vi "Score Particles.vi"(8 "Area Size Limit":i32=444, 9 "Particle Count Limit":i32=10, 11 "Image Refnum in":T2) -> (0 "Size Array":T1(array[cluster]), 2 "Scored Particle Info":T3(array[cluster]), 3 "Image Refnum out":T2)   [LabVIEW 2011]
doc: "Score the largest particles in the image to determine how well they match the target attributes. Specifically, calculate how rectangular a particle is, inspect its aspect ratio, and determine if it is hollow (having pixels on around the edges, but off in the large center)."
uses:
  <vilib>/vision/Image Controls.llb/IMAQ Image.ctl
  <vilib>/vision/NI_Vision_Development_Module.lvlib
panel:
  out "Bounding Height":dbl
  out "Bounding Width":dbl
  out "Area":dbl
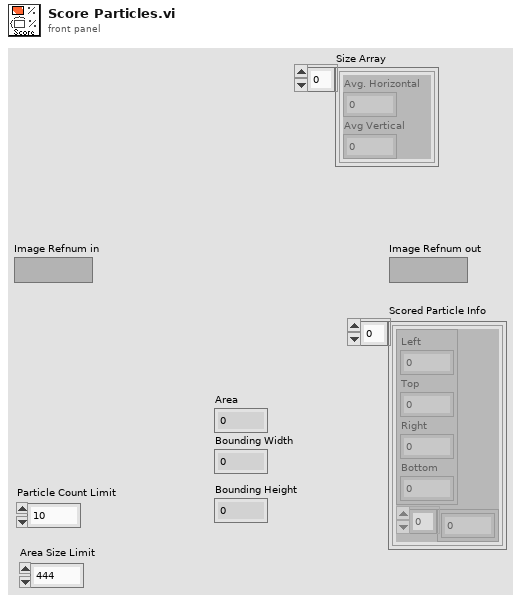
[diagram p1: front panel]
types:
  T1 = cluster{"Avg. Horizontal ":dbl, "Avg Vertical":dbl}[]
  T2 = typedef "IMAQ Image.ctl" = refnum<image>
  T3 = cluster{cluster{"Left":dbl, "Top":dbl, "Right":dbl, "Bottom":dbl}, dbl[]}[]
  T4 = typedef "Particle Parameters" = i32
  T5 = typedef "Image Type" = u32
  T6 = cluster{"Left":dbl, "Top":dbl, "Right":dbl, "Bottom":dbl}
  T7 = cluster{cluster{"Left":dbl, "Top":dbl, "Right":dbl, "Bottom":dbl}, dbl[]}
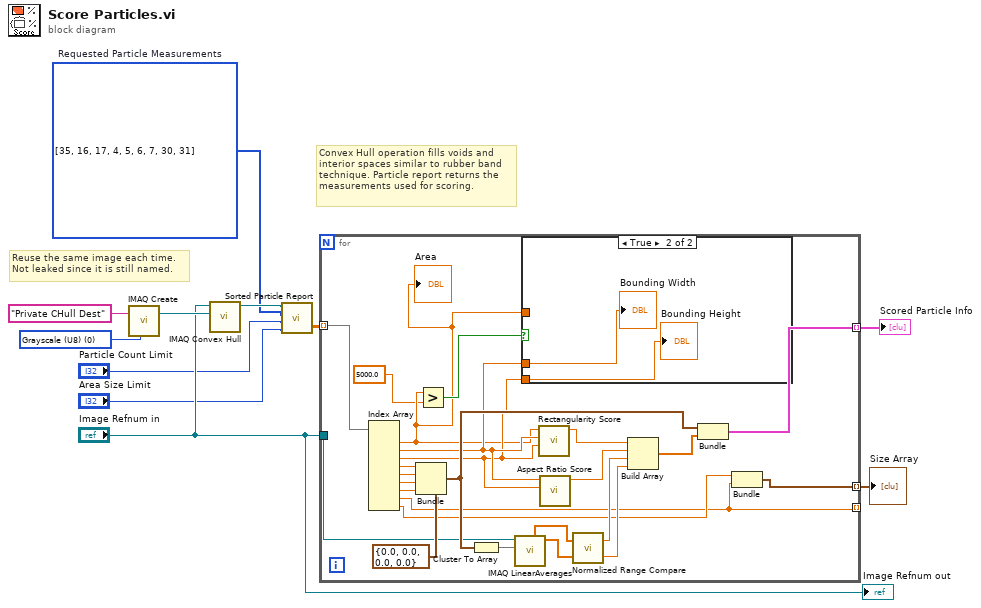
[diagram p0: block diagram]
diagram:
  w2 = T4[] [35, 16, 17, 4, 5, 6, 7, 30, 31] items=["Center of Mass X", "Center of Mass Y", "First Pixel X", "First Pixel Y", "Bounding Rect Left", "Bounding Rect Top", "Bounding Rect Right", "Bounding Rect Bottom", "Max Feret Diameter Start X", "Max Feret Diameter Start Y", "Max Feret Diameter End X", "Max Feret Diameter End Y", "Max Horiz. Segment Length Left", "Max Horiz. Segment Length Right", "Max Horiz. Segment Length Row", "-", "Bounding Rect Width", "Bounding Rect Height", "Bounding Rect Diagonal", "Perimeter", "Convex Hull Perimeter", "Holes' Perimeter", "Max Feret Diameter", "Equivalent Ellipse Major Axis", "Equivalent Ellipse Minor Axis", "Equivalent Ellipse Minor Axis (Feret)", "Equivalent Rect Long Side", "Equivalent Rect Short Side", "Equivalent Rect Diagonal", "Equivalent Rect Short Side (Feret)", "Average Horiz. Segment Length", "Average Vert. Segment Length", "Hydraulic Radius", "Waddel Disk Diameter", "-", "Area", "Holes' Area", "Particle & Holes' Area", "Convex Hull Area", "Image Area", "-", "Number of Holes", "Number of Horiz. Segments", "Number of Vert. Segments", "-", "Orientation", "Max Feret Diameter Orientation", "-", "% Area/Image Area", "% Area/(Particle & Holes' Area)", "Ratio of Equivalent Ellipse Axes", "Ratio of Equivalent Rect Sides", "-", "Elongation Factor", "Compactness Factor", "Heywood Circularity Factor", "Type Factor", "-", "Sum X", "Sum Y", "Sum XX", "Sum XY", "Sum YY", "Sum XXX", "Sum XXY", "Sum XYY", "Sum YYY", "-", "Moment of Inertia XX", "Moment of Inertia XY", "Moment of Inertia YY", "Moment of Inertia XXX", "Moment of Inertia XXY", "Moment of Inertia XYY", "Moment of Inertia YYY", "Norm. Moment of Inertia XX", "Norm. Moment of Inertia XY", "Norm. Moment of Inertia YY", "Norm. Moment of Inertia XXX", "Norm. Moment of Inertia XXY", "Norm. Moment of Inertia XYY", "Norm. Moment of Inertia YYY", "Hu Moment 1", "Hu Moment 2", "Hu Moment 3", "Hu Moment 4", "Hu Moment 5", "Hu Moment 6", "Hu Moment 7"]  # Requested Particle Measurements
  w9 = T5 0 items=["Grayscale (U8)", "Grayscale (I16)", "Grayscale (SGL)", "Complex (CSG)", "RGB (U32)", "HSL (U32)", "RGB (U64)", "Grayscale (U16)"] ("Image Type")
  # "Reuse the same image each time.\nNot leaked since it is still named."
  # "Convex Hull operation fills voids and\ninterior spaces similar to rubber band\ntechnique. Particle report returns the\nmeasurements used for scoring."
  n1 = call "IMAQ Create"("Image Name"="Private CHull Dest", "Image Type"=w9) -> ("New Image"=w8:T2)  [unwired: 2 in, 2 out]
  n2 = call "IMAQ Convex Hull"("Image Dst"=w8, "Image Src"="Image Refnum in") -> ("Image Dst Out"=w6:T2)  [unwired: 2 in, 7 out]
  n3 = call "Sorted Particle Report.vi"("Area Size Limit"="Area Size Limit", "Particle Count Limit"="Particle Count Limit", "Pixel Measurements"=w2, "Image in"=w6) -> ("Sorted Data"=w3:dbl[][])  [unwired: 1 out]
  n4 = for {
    tunnel: [w35] -> w11 mode=indexing
    tunnel: "Image Refnum in" -> [w31]
    tunnel: w3 -> [w30] mode=indexing
    tunnel: [w13] -> _ mode=indexing
    tunnel: [w12] -> w1 mode=indexing
    n5 = Index Array(array=w30) -> (element #1=w16:dbl, element #2=w18:dbl, element #3=w17:dbl, element #4=w26:dbl, element #5=w27:dbl, element #6=w28:dbl, element #7=w29:dbl, element #8=w13:dbl, element #9=w14:dbl)  [unwired: 9 in]
    "Area" <- w16
    n6 = Bundle(cluster=T6 {"Left"=0.0, "Top"=0.0, "Right"=0.0, "Bottom"=0.0}, "Left"=w26, "Top"=w27, "Right"=w28, "Bottom"=w29) -> (w34:T6)
    n7 = Greater?(x=w16, y=5000.0 ("x")) -> (0:w19:bool)
    n8 = Cluster To Array(cluster=w34) -> (array=w32:dbl[])
    n9 = call "IMAQ LinearAverages"("Optional Rectangle"=w32, "Image Src"=w31) -> ("Y Axis Averages"=w23:sgl[], "X Axis Averages"=w22:sgl[])  [unwired: 2 in, 6 out]
    n10 = case shown="True" w19 {
      tunnel: w16 -> [_ _]
      tunnel: w18 -> [_ w38]
      tunnel: w17 -> [_ w37]
      frame False {
      }
      frame True {
        "Bounding Width" <- w38
        "Bounding Height" <- w37
      }
    }
    n11 = call "Rectangularity Score.vi"("Height"=w17, "Width"=w18, "Area"=w16) -> ("Score"=w25:dbl)  [unwired: 8 in]
    n12 = call "Aspect Ratio Score.vi"("Height"=w17, "Width"=w18) -> ("Score"=w24:dbl)  [unwired: 9 in]
    n13 = call "Normalized Range Compare.vi"("Y Averages"=w23, "X Averages"=w22) -> ("Y Score"=w20:dbl, "X Score"=w21:dbl)
    n14 = Build Array(w25, w24, w21, w20) -> (w33:dbl[])
    n15 = Bundle(w34, w33) -> (w35:T7)  [unwired: 1 in]
    n16 = Bundle("Numeric"=w14, "Numeric"=w13) -> (w12:cluster{"Numeric":dbl, "Numeric":dbl})  [unwired: 1 in]
  }
  "Scored Particle Info" <- w11
  "Size Array" <- w1
  "Image Refnum out" <- "Image Refnum in"
